vi "FT_sensor_tester_stream old.vi"() -> ()   [LabVIEW 2018]
uses:
  <vilib>/Analysis/baseanly.llb/Mean (DBL).vi
  <vilib>/Analysis/baseanly.llb/A x Vector.vi
  <vilib>/Analysis/NI_AALBase.lvlib
  <vilib>/ptbypt/NI_PtbyPt.lvlib
panel:
  out "Execution ms":dbl format="%0.2f"
  out "Sample rate (Hz)":dbl format="%0.2f"
  out "Array":dbl[](array[numeric])
  out "Data":T1
  in  "Stop Stream":bool
  out "Waveform Chart":T2(graph)
  in  "Start Stream":bool
  out "Error Code":T3(ring)
  out "Return FID":u8=2
  out "FID":u8=2
  in  "IP Address":string="192.168.5.101"
  out "error out":errorcluster={"status"=TRUE, "code"=56, "source"="TCP Open Connection in FT_sensor_tester_stream.vi"}
  in  "Stop":bool
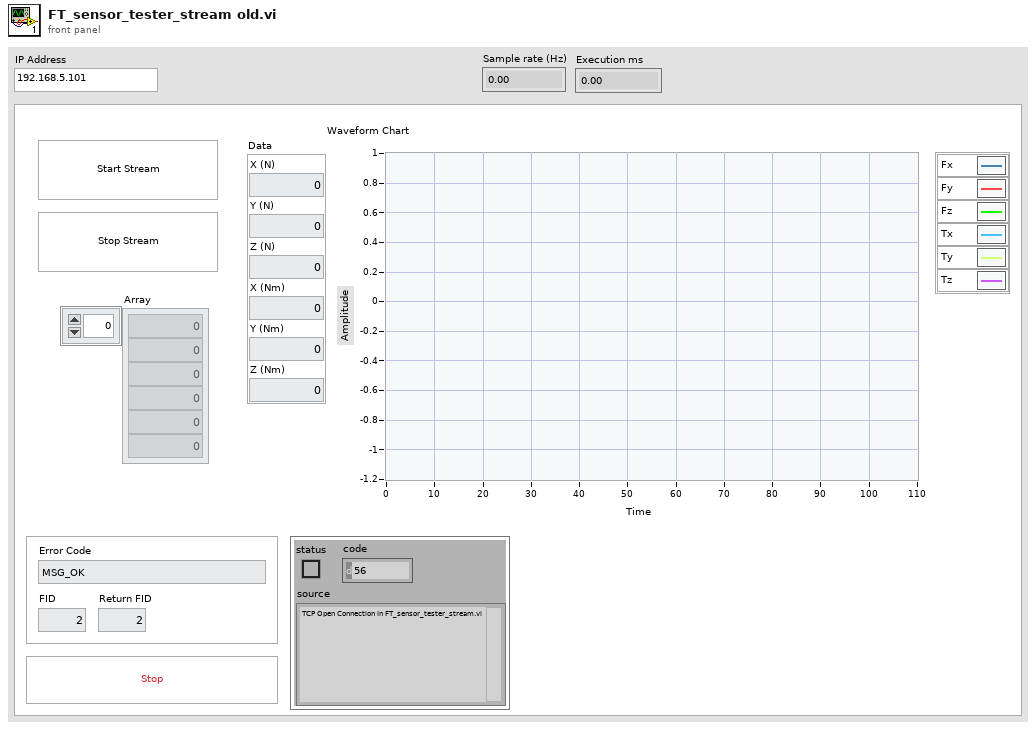
[diagram p1: front panel]
types:
  T1 = cluster{"X (N)":dbl, "Y (N)":dbl, "Z (N)":dbl, "X (Nm)":dbl, "Y (Nm)":dbl, "Z (Nm)":dbl}
  T2 = cluster{"[0]":dbl, "[1]":dbl, "[2]":dbl, "[3]":dbl, "[4]":dbl, "[5]":dbl, "[6]":dbl, "[7]":dbl, "[8]":dbl}
  T3 = enum8{"MSG_OK", "MSG_ERROR_NOT_SUPPORTED", "MSG_ERROR_SENSOR_DISCONNECTED", "MSG_ERROR_READING_PENDING"}
  T4 = cluster{"[0]":dbl, "[1]":dbl, "[2]":dbl, "[3]":dbl, "[4]":dbl, "[5]":dbl, "[6]":dbl, "[7]":dbl, "[8]":dbl}[]
  T5 = enum16{"Default", "Start Acquisition Stream", "Stop Acquisition Stream", "Read"}
  T6 = enum16{"big-endian, network order", "native, host order", "little-endian"}
  T7 = cluster{"pumpState":i32, "suppliedVolume_ml":sgl, "flowRate_mlmin":sgl, "home":i32, "port":i32}
  T8 = cluster{"connection ID":refnum<k5>, "header length":u16}
  T9 = cluster{"header":cluster{"length":u16, "fid":u8, "error":u8}}
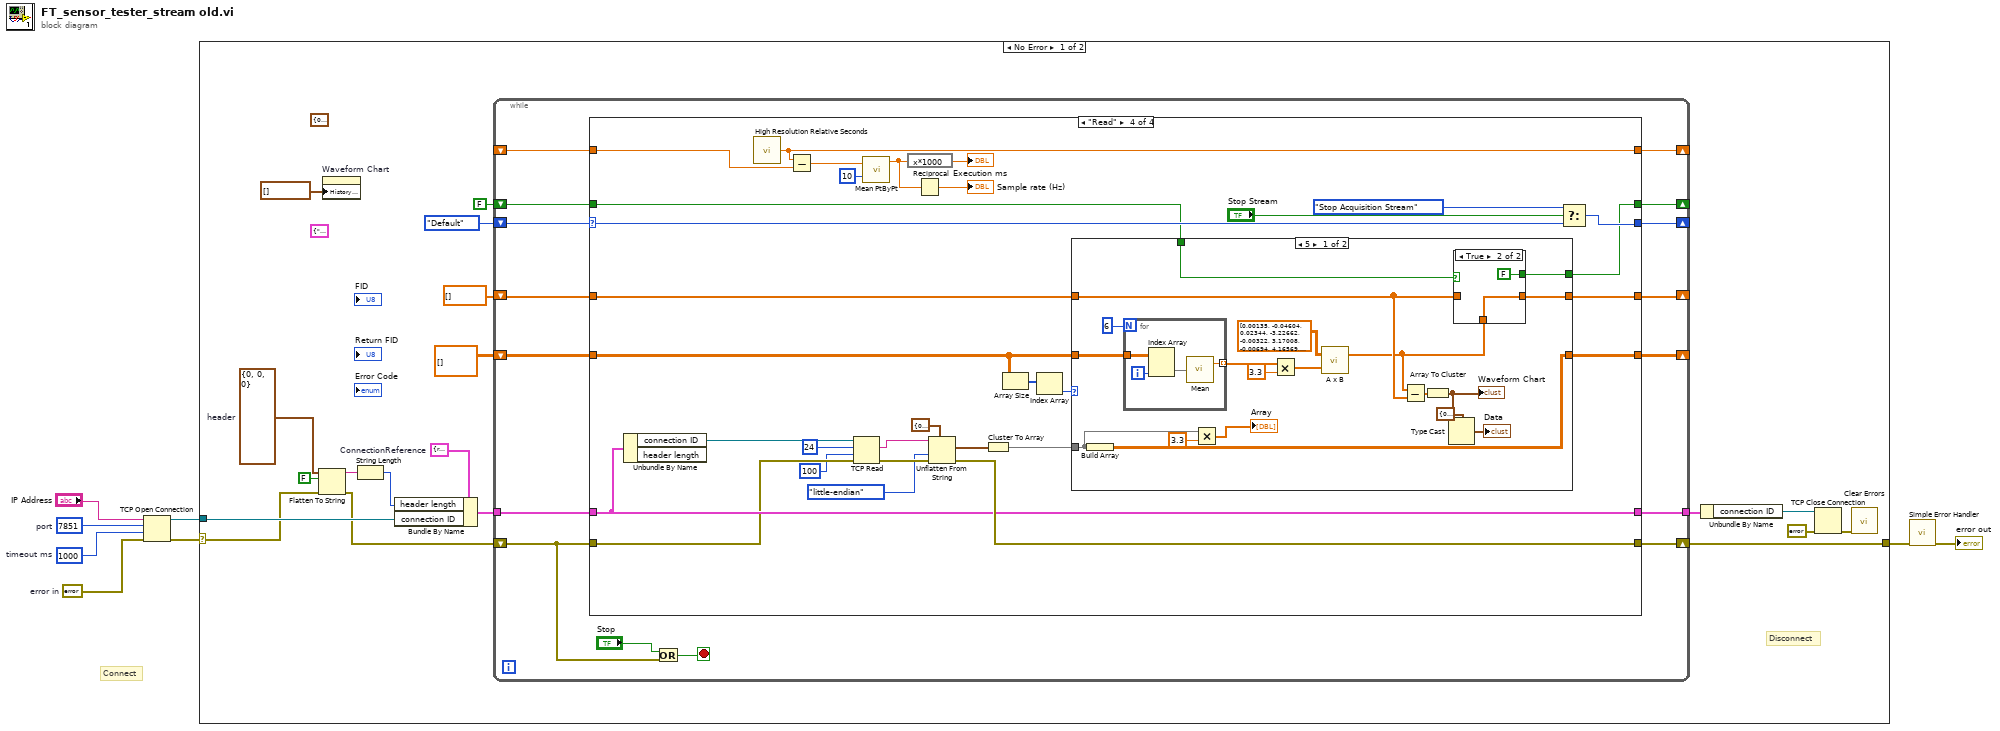
[diagram p0: block diagram]
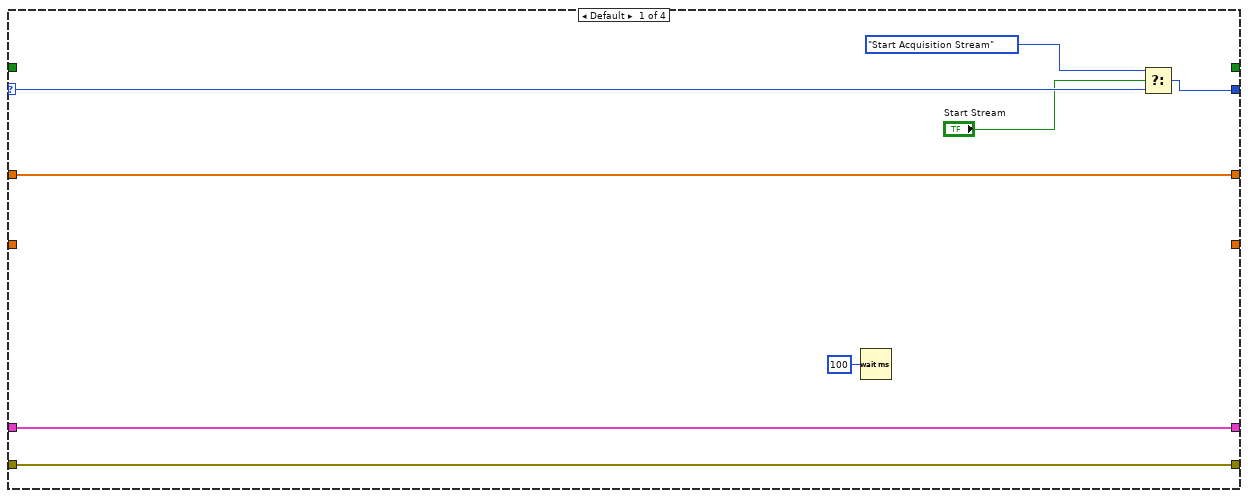
[diagram p2: hidden frame]
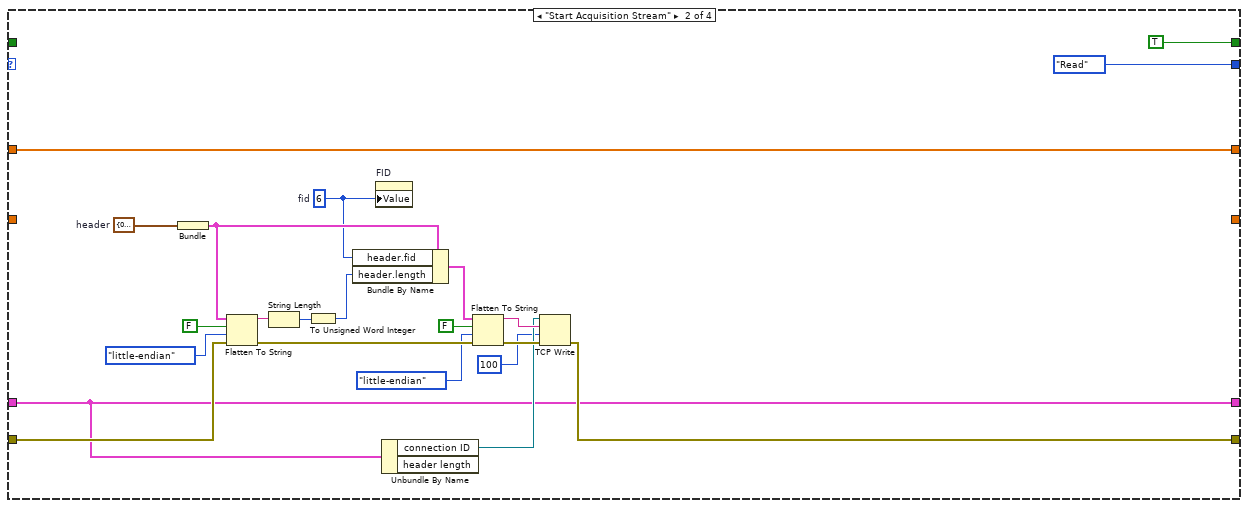
[diagram p3: hidden frame]
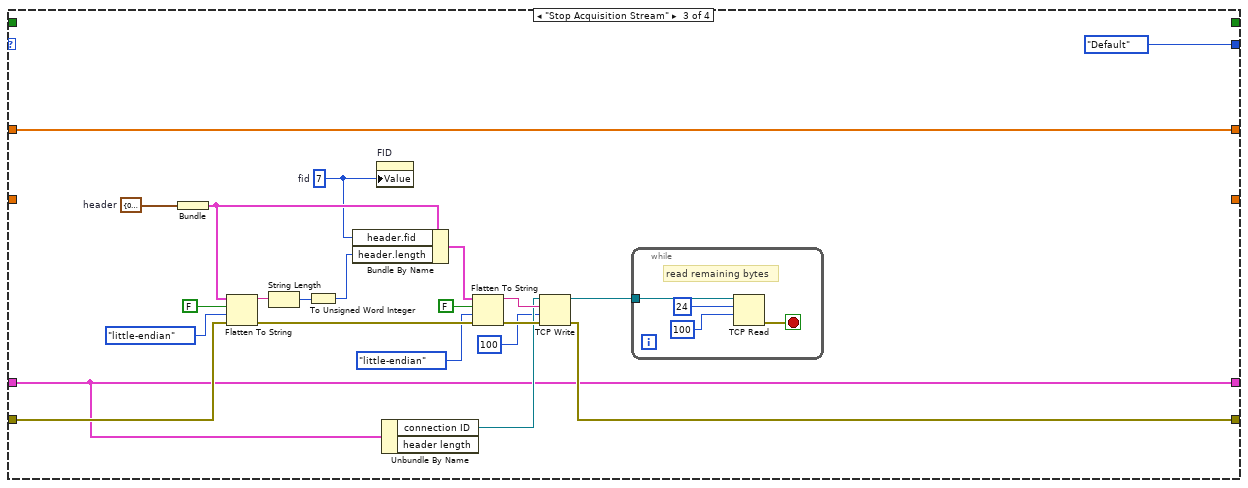
[diagram p4: hidden frame]
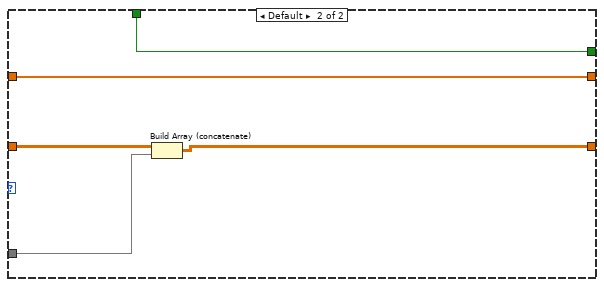
[diagram p6: hidden frame]
diagram:
  w6 = errorcluster {"status"=FALSE, "code"=0, "source"=""}  # error in
  w7 = 1000  # timeout ms
  w8 = u16 7851  # port
  # "Connect"
  n1 = TCP Open Connection(address="IP Address", remote port or service name=w8, timeout ms (60000)=w7, error in (no error)=w6) -> (connection ID=w5:refnum<k5>, error out=w1:errorcluster)  [unwired: 1 in]
  n2 = case shown="No Error" w1 {
    selector: w1 -> [w16 w162]
    tunnel: w5 -> [w23 _]
    tunnel: [w14 w162] -> w2
    frame No Error {
      (unwired) cluster{"axis":string, "stepPeriod (ms)":string} {"axis"="", "stepPeriod (ms)"=""} ("Return Motor Config")
      (unwired) T7 {"pumpState"=0, "suppliedVolume_ml"=0.0, "flowRate_mlmin"=0.0, "home"=0, "port"=0} ("Status")
      w22 = cluster{"length":u16, "fid":u8, "error":u8} {"length"=0, "fid"=0, "error"=0}  # header
      w24 = T8 {"connection ID"=refnum, "header length"=0}  # ConnectionReference
      # "Disconnect"
      n3 = Flatten To String(anything=w22, prepend array or string size? (T)=FALSE, error in (no error)=w16) -> (data string=w20:string, error out=w17:errorcluster)  [unwired: 1 in, 1 out]
      n4 = property on="Waveform Chart" class="WFChart (strict)"("History Data"=T4 []) -> ()  [unwired: 2 in, 2 out]
      n5 = String Length(string=w20) -> (length=w19:i32)
      n6 = Bundle By Name(cluster=w24, "header length"=w19, "connection ID"=w23) -> (w18:T8)
      n7 = while {
        tunnel: w18 -> [w38]
        shift-right: [w40] -> w14
        shift-left: w17 -> [w41]
        tunnel: [w39] -> w15
        shift-right: [w37] -> _
        shift-left: T5."Default" ("Case") -> [w36]
        shift-right: [w35] -> _
        shift-left: sgl[][] [] ("appended array") -> [w34]
        shift-right: [w33] -> _
        shift-left: dbl[] [] ("A x Vector") -> [w32]
        shift-right: [w31] -> _
        shift-left: FALSE -> [w30]
        shift-right: [w29] -> _
        shift-left: _ -> [w28]
        stop <- w43 stop-if-true
        n8 = case shown="\"Read\"" w36 {
          selector: w36 -> [w51 _ _ w121]
          tunnel: w41 -> [w45 w58 w80 w122]
          tunnel: [w45 w57 w79 w127] -> w40
          tunnel: [w46 w56 w78 w126] -> w39
          tunnel: w38 -> [w46 w56 w78 w126]
          tunnel: [w49 T5."Read" ("Case") T5."Default" ("t") w123] -> w37
          tunnel: [_ _ _ w120] -> w35
          tunnel: w34 -> [_ _ _ w116]
          tunnel: [w44 w53 w75 w110] -> w33
          tunnel: w32 -> [w44 w53 w75 w109]
          tunnel: [_ TRUE _ w107] -> w31
          tunnel: w30 -> [_ _ _ w108]
          tunnel: [_ _ _ w105] -> w29
          tunnel: w28 -> [_ _ _ w106]
          frame Default {
            n9 = Wait (ms)(milliseconds to wait=u32 100) -> ()  [unwired: 1 out]
            n10 = Select(t=T5."Start Acquisition Stream", s="Start Stream", f=w51) -> (s? t:f=w49:T5)
          }
          frame "Start Acquisition Stream" {
            w63 = cluster{"length":u16, "fid":u8, "error":u8} {"length"=0, "fid"=0, "error"=0}  # header
            w55 = u8 6  # fid
            n11 = Bundle("header"=w63) -> (w69:T9)  [unwired: 1 in]
            n12 = Flatten To String(anything=w69, prepend array or string size? (T)=FALSE, byte order (0:big-endian, network order)=T6."little-endian", error in (no error)=w58) -> (data string=w67:string, error out=w68:errorcluster)  [unwired: 1 out]
            n13 = String Length(string=w67) -> (length=w66:i32)
            n14 = To Unsigned Word Integer(number=w66) -> (unsigned 16bit integer=w65:u16)
            n15 = Bundle By Name(cluster=w69, "header.fid"=w55, "header.length"=w65) -> (w70:T9)
            n16 = property on="FID" class="DigNum (strict)"("Value"=w55) -> ()  [unwired: 2 in, 2 out]
            n17 = Unbundle By Name(w56) -> ("connection ID"=w61:refnum<k5>)  [unwired: 1 out]
            n18 = Flatten To String(anything=w70, prepend array or string size? (T)=FALSE, byte order (0:big-endian, network order)=T6."little-endian", error in (no error)=w68) -> (data string=w72:string, error out=w73:errorcluster)  [unwired: 1 out]
            n19 = TCP Write(connection ID=w61, data in=w72, error in (no error)=w73, 9:100 ("timeout ms (25000)")) -> (error out=w57:errorcluster)  [unwired: 2 out]
          }
          frame "Stop Acquisition Stream" {
            w85 = cluster{"length":u16, "fid":u8, "error":u8} {"length"=0, "fid"=0, "error"=0}  # header
            w77 = u8 7  # fid
            n20 = Bundle("header"=w85) -> (w91:T9)  [unwired: 1 in]
            n21 = Flatten To String(anything=w91, prepend array or string size? (T)=FALSE, byte order (0:big-endian, network order)=T6."little-endian", error in (no error)=w80) -> (data string=w89:string, error out=w90:errorcluster)  [unwired: 1 out]
            n22 = String Length(string=w89) -> (length=w88:i32)
            n23 = To Unsigned Word Integer(number=w88) -> (unsigned 16bit integer=w87:u16)
            n24 = Bundle By Name(cluster=w91, "header.fid"=w77, "header.length"=w87) -> (w92:T9)
            n25 = property on="FID" class="DigNum (strict)"("Value"=w77) -> ()  [unwired: 2 in, 2 out]
            n26 = Unbundle By Name(w78) -> ("connection ID"=w83:refnum<k5>)  [unwired: 1 out]
            n27 = Flatten To String(anything=w92, prepend array or string size? (T)=FALSE, byte order (0:big-endian, network order)=T6."little-endian", error in (no error)=w90) -> (data string=w94:string, error out=w95:errorcluster)  [unwired: 1 out]
            n28 = TCP Write(connection ID=w83, data in=w94, error in (no error)=w95, 9:100 ("timeout ms (25000)")) -> (connection ID out=w74:refnum<k5>, error out=w79:errorcluster)  [unwired: 1 out]
            n29 = while {
              tunnel: w74 -> [w97]
              stop <- w96 stop-if-true
              # "read remaining bytes"
              n30 = TCP Read(connection ID=w97, bytes to read=24, 9:100 ("timeout ms (25000)")) -> (error out=w96:errorcluster)  [unwired: 2 in, 2 out]
            }
          }
          frame "Read" {
            n31 = Unbundle By Name(w126) -> ("connection ID"=w130:refnum<k5>)  [unwired: 1 out]
            n32 = call <vilib>:"High Resolution Relative Seconds.vi"() -> ("relative seconds"=w105:dbl)
            n33 = Subtract(x=w105, y=w106) -> (x-y=w103:dbl)
            n34 = TCP Read(connection ID=w130, bytes to read=24, error in (no error)=w122, 9:100 ("timeout ms (25000)")) -> (data out=w113:string, error out=w129:errorcluster)  [unwired: 1 in, 1 out]
            n35 = call <vilib>:"Mean PtByPt.vi"("x"=w103, "sample length"=10) -> ("mean"=w101:dbl)  [unwired: 2 in, 1 out]
            n36 = expression code="x*1000"(w101) -> (→"Execution ms":dbl)
            n37 = Reciprocal(x=w101) -> (1/x=→"Sample rate (Hz)":dbl)
            n38 = Unflatten From String(type=cluster{sgl, sgl, sgl, sgl, sgl, sgl} {0.0, 0.0, 0.0, 0.0, 0.0, 0.0}, binary string=w113, byte order (0:big-endian, network order)=T6."little-endian", error in (no error)=w129) -> (value=w118:cluster{sgl, sgl, sgl, sgl, sgl, sgl}, error out=w127:errorcluster)  [unwired: 1 in, 1 out]
            n39 = Cluster To Array(cluster=w118) -> (array=w117:sgl[])
            n40 = Array Size(array=w116) -> (size(s)=w115:i32[])
            n41 = Index Array(array=w115) -> (element=w114:i32)  [unwired: 1 in]
            n42 = case shown="5" w114 {
              tunnel: w116 -> [w143 w159]
              tunnel: [w144 w160] -> w120
              tunnel: w117 -> [w132 w161]
              tunnel: [w149 w158] -> w110
              tunnel: w109 -> [w148 w158]
              tunnel: w108 -> [w146 w157]
              tunnel: [w145 w157] -> w107
              frame 5 {
                n43 = Build Array(w132) -> (w144:sgl[][])
                n44 = for {
                  N: 6 -> [_]
                  tunnel: w143 -> [w152]
                  tunnel: [w153] -> w135 mode=indexing
                  i -> [w151]
                  n45 = Index Array(array=w152, index (col)=w151) -> (element=w150:sgl[])  [unwired: 1 in]
                  n46 = call-poly <vilib>:"Mean.vi"("X"=w150) -> ("mean"=w153:dbl)  [unwired: 1 out]
                }
                n47 = Multiply ("Multiply.vi")(x=w132, y=3.3) -> (x*y=→"Array":dbl[])
                n48 = Multiply ("Multiply.vi")(x=w135, y=3.3) -> (x*y=w134:dbl[])
                n49 = call-poly <vilib>:"A x B.vi"("Vector"=w134, "A"=dbl[][] [[0.00135, -0.04604, 0.02344, -3.22662, -0.00322, 3.17008], [-0.00694, 4.16569, 0.02971, -1.87643, 0.02738, -1.79608], [3.69182, 0.02713, 3.83425, -0.03329, 3.65801, -0.067], [0.15408, 25.37956, 21.34115, -11.71178, -20.50426, -10.51265], [-23.9405, 0.07684, 12.2178, 19.58172, 12.22442, -19.60731], [0.09832, 17.49271, -0.32435, 15.76607, -0.09154, 15.24495]] ("Calibration Matrix")) -> ("A x Vector"=w136:dbl[])  [unwired: 1 out]
                n50 = Subtract(x=w136, y=w148) -> (x-y=w142:dbl[])
                n51 = Array To Cluster(array=w142) -> (cluster=w140:T2)
                "Waveform Chart" <- w140
                n52 = Type Cast(type=T1 {"X (N)"=0.0, "Y (N)"=0.0, "Z (N)"=0.0, "X (Nm)"=0.0, "Y (Nm)"=0.0, "Z (Nm)"=0.0} ("Data"), x=w140) -> (*(type *) &x=→"Data":T1)
                n53 = case shown="True" w146 {
                  tunnel: [w154 w156] -> w149
                  tunnel: w136 -> [_ w156]
                  tunnel: w148 -> [w154 _]
                  tunnel: [_ FALSE] -> w145
                  frame False {
                  }
                  frame True {
                  }
                }
              }
              frame Default {
                n54 = Build Array (concatenate)(w159, w161) -> (w160:sgl[][])
              }
            }
            n55 = Select(t=T5."Stop Acquisition Stream", s="Stop Stream", f=w121) -> (s? t:f=w123:T5)
          }
        }
        n56 = Or(x="Stop", y=w41) -> (x .or. y?=w43:bool)
      }
      n57 = Unbundle By Name(w15) -> ("connection ID"=w25:refnum<k5>)
      n58 = TCP Close Connection(connection ID=w25, error in (no error)=errorcluster {"status"=FALSE, "code"=0, "source"=""}) -> (error out=w26:errorcluster)  [unwired: 1 in, 1 out]
      n59 = call <vilib>:"Clear Errors.vi"("error in (no error)"=w26) -> ()  [unwired: 5 in, 2 out]
    }
    frame Error {
    }
  }
  n60 = call <vilib>:"Simple Error Handler.vi"("error in (no error)"=w2) -> ("error out"=→"error out":errorcluster)  [unwired: 4 in, 4 out]
